vi "Create String Picture.vi"(11 "string":string) -> (3 "string picture":picture)   [LabVIEW 2017]
doc: "Converts <b>string</b> into <b>string picture</b> using custom font (Default Settings.vi:font)."
uses:
  Settings/Default Settings.vi
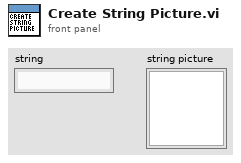
[diagram p1: front panel]
types:
  T1 = typedef "imagedata.ctl" = cluster{"image type":i32, "image depth":i32, "image":u8[], "mask":u8[], "colors":u32[], "Rectangle":cluster{"left":i16, "top":i16, "right":i16, "bottom":i16}}
  T2 = cluster{"left":i16, "top":i16, "right":i16, "bottom":i16}
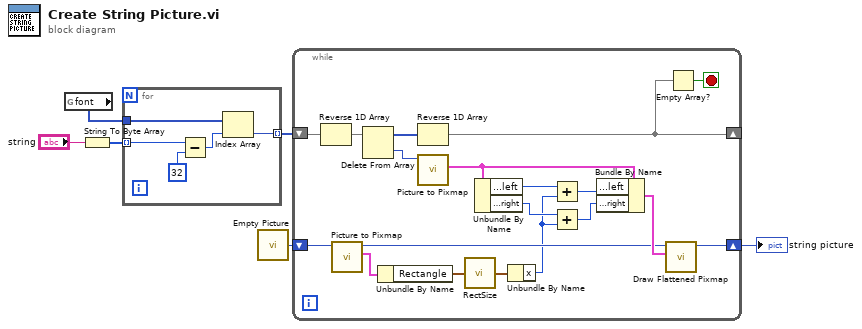
[diagram p0: block diagram]
diagram:
  n1 = global read "Default Settings.vi" "font"() -> (w1:picture[])
  n2 = String To Byte Array(string="string") -> (unsigned byte array=w2:u8[])
  n3 = for {
    tunnel: w2 -> [w11] mode=indexing
    tunnel: [w8] -> w5 mode=indexing
    tunnel: w1 -> [w7]
    n4 = Subtract(x=w11, y=u8 32) -> (x-y=w9:u8)
    n5 = Index Array(array=w7, index=w9) -> (element=w8:picture)
  }
  n6 = call "Empty Picture"() -> ("empty picture"=w4:picture)
  n7 = while {
    shift-right: [w29] -> _
    shift-left: w5 -> [w30]
    shift-right: [w18] -> w6
    shift-left: w4 -> [w27]
    stop <- w28 stop-if-true
    n8 = Reverse 1D Array(array=w30) -> (reversed array=w14:picture[])
    n9 = call <vilib>:"Picture to Pixmap.vi"("picture"=w27) -> ("image data"=w26:T1, "new picture"=w19:picture)  [unwired: 9 in]
    n10 = Delete From Array(array=w14) -> (deleted portion=w12:picture, array with subset deleted=w13:picture[])  [unwired: 2 in]
    n11 = Unbundle By Name(w26) -> ("Rectangle"=w17:T2)
    n12 = Reverse 1D Array(array=w13) -> (reversed array=w29:picture[])
    n13 = call <vilib>:"Picture to Pixmap.vi"("picture"=w12) -> ("image data"=w25:T1)  [unwired: 9 in, 1 out]
    n14 = call <vilib>:"RectSize.vi"("rect"=w17) -> ("point"=w16:cluster{"x":i16, "y":i16})
    n15 = Unbundle By Name(w25) -> ("Rectangle.left"=w24:i16, "Rectangle.right"=w22:i16)
    n16 = Unbundle By Name(w16) -> ("x"=w15:i16)
    n17 = Add(x=w24, y=w15) -> (x+y=w23:i16)
    n18 = Add(x=w22, y=w15) -> (x+y=w21:i16)
    n19 = Bundle By Name(cluster=w25, "Rectangle.left"=w23, "Rectangle.right"=w21) -> (w20:T1)
    n20 = call <vilib>:"Draw Flattened Pixmap.vi"("image data"=w20, "picture"=w19) -> ("new picture"=w18:picture)  [unwired: 7 in]
    n21 = Empty Array?(array=w29) -> (empty?=w28:bool)
  }
  "string picture" <- w6
